vi "Fit.vi"(11 "ExpFitter in":refnum<class "ExpFitter.lvclass">) -> (3 "ExpFitter out":refnum<class "ExpFitter.lvclass">)   [LabVIEW 2019, in "ExpFitter.lvclass"]
uses:
  ExpFitter.lvclass
  ExpFitter.lvclass/ExpFitter.ctl
  <vilib>/Analysis/NI_AALPro.lvlib
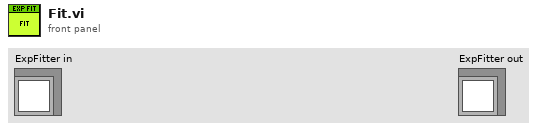
[diagram p1: front panel]
types:
  T1 = cluster{"amp min":dbl, "amp max":dbl, "damping min":dbl, "damping max":dbl, "offset min":dbl, "offset max":dbl}
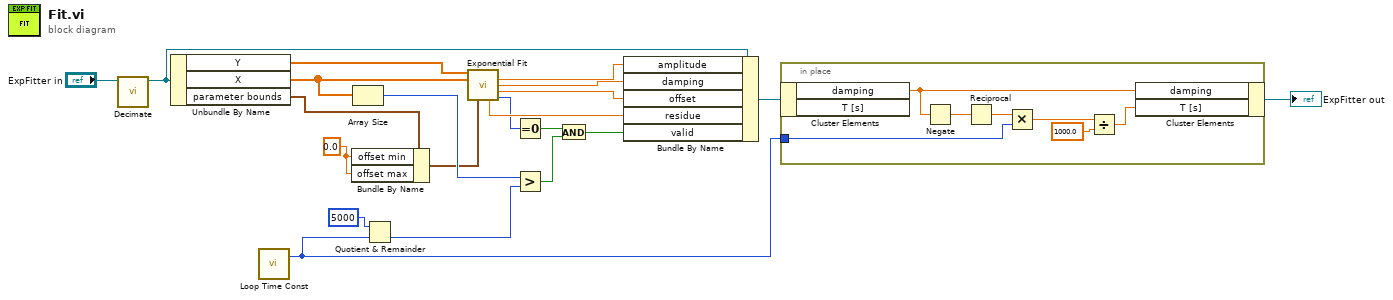
[diagram p0: block diagram]
diagram:
  w1 = 0.0 ("offset max")
  n1 = call "Decimate.vi"("ExpFitter in"="ExpFitter in") -> ("ExpFitter out"=w14:refnum<class "ExpFitter.lvclass">)  [unwired: 9 in, 1 out]
  n2 = Unbundle By Name(w14) -> ("Y"=w21:dbl[], "X"=w7:dbl[], "parameter bounds"=w20:T1)
  n3 = call "Loop Time Const.vi"() -> ("loop time ms"=w3:i64)  [unwired: 3 in]
  n4 = Bundle By Name(cluster=w20, "offset min"=w1, "offset max"=w1) -> (w2:T1)
  n5 = Array Size(array=w7) -> (size(s)=w6:i32)
  n6 = Quotient & Remainder(x=i64 5000, y=w3) -> (floor(x/y)=w10:i64)  [unwired: 1 out]
  n7 = call <vilib>:"Exponential Fit.vi"("Y"=w21, "X"=w7, "parameter bounds"=w2) -> ("amplitude"=w19:dbl, "damping"=w18:dbl, "offset"=w17:dbl, "residue"=w16:dbl, "error"=w12:i32)  [unwired: 7 in, 1 out]
  n8 = Equal To 0?(x=w12) -> (x = 0?=w13:bool)
  n9 = Greater?(x=w6, y=w10) -> (0:w8:bool)
  n10 = And(x=w13, y=w8) -> (x .and. y?=w9:bool)
  n11 = Bundle By Name(cluster=w14, "amplitude"=w19, "damping"=w18, "offset"=w17, "residue"=w16, "valid"=w9) -> (w5:refnum<class "ExpFitter.lvclass">)
  n12 = in-place {
    in-place-border: w3 -> [w26]
    n13 = in-place-cluster #1(w5) -> ("damping"=w22:dbl)  [unwired: 1 out]
    n14 = Negate(x=w22) -> (-x=w28:dbl)
    n15 = Reciprocal(x=w28) -> (1/x=w27:dbl)
    n16 = Multiply(x=w27, y=w26) -> (x*y=w25:dbl)
    n17 = Divide(x=w25, y=1000.0) -> (x/y=w23:dbl)
    n18 = in-place-cluster #1("damping"=w22, "T [s]"=w23) -> (→"ExpFitter out":refnum<class "ExpFitter.lvclass">)
  }
